vi "dotNET SSL Socket.vi"() -> ()   [LabVIEW 2013]
uses:
  dotNET SSL Socket/dotNET SSL Server/dotNET SSL Server.lvclass
  dotNET SSL Socket/dotNET SSL Listener/dotNET Listener.lvclass
panel:
  out "error out":errorcluster
  in  "stop":bool
  out "string":string
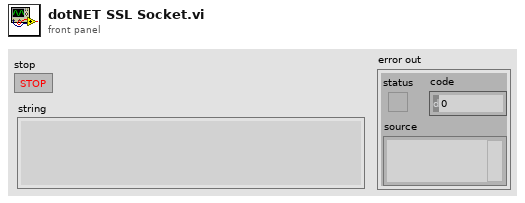
[diagram p1: front panel]
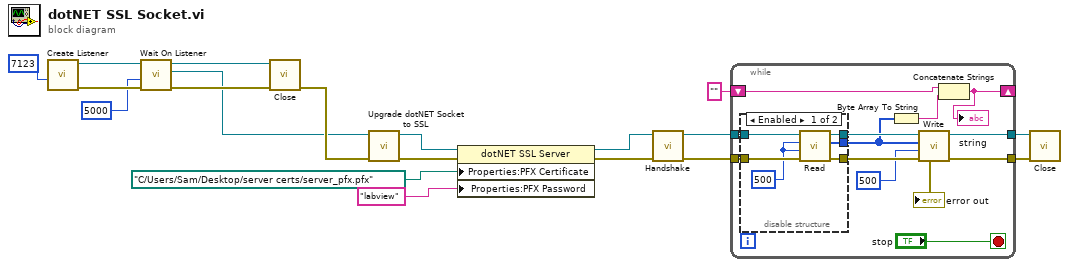
[diagram p0: block diagram]
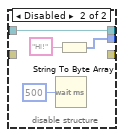
[diagram p2: hidden frame]
diagram:
  n1 = call-dynamic "Create Listener.vi"("timeout ms (5000)"=7123 ("port")) -> ("error out"=w15:errorcluster, "dotNET Listener out"=w14:refnum<class "dotNET Listener.lvclass">)  [unwired: 9 in]
  n2 = call-dynamic "Wait On Listener.vi"("error in (no error)"=w15, "timeout ms (5000)"=5000, "dotNET Listener in"=w14) -> ("error out"=w11:errorcluster, "Socket out"=w3:refnum<class "Socket.lvclass">, "dotNET Listener out"=w13:refnum<class "dotNET Listener.lvclass">)  [unwired: 6 in]
  n3 = call-dynamic "Close.vi"("error in (no error)"=w11, "dotNET Listener in"=w13) -> ("error out"=w10:errorcluster)  [unwired: 9 in]
  n4 = call "Upgrade dotNET Socket to SSL.vi"("error in (no error)"=w10, "Socket in"=w3) -> ("error out"=w9:errorcluster, "dotNET SSL Socket out"=w7:refnum<class "dotNET SSL Server.lvclass">)  [unwired: 8 in]
  n5 = property class="dotNET SSL Server"(reference=w7, error in=w9, "Properties:PFX Certificate"=path "C:/Users/Sam/Desktop/server certs/server_pfx.pfx", "Properties:PFX Password"="labview" ("password")) -> (reference out=w6:refnum<class "dotNET SSL Server.lvclass">, error out=w8:errorcluster)
  n6 = call-dynamic "Handshake.vi"("error in (no error)"=w8, "dotNET SSL Socket in"=w6) -> ("error out"=w2:errorcluster, "dotNET SSL Socket out"=w1:refnum<class "dotNET SSL Server.lvclass">)  [unwired: 8 in]
  n7 = while {
    tunnel: w2 -> [w31]
    tunnel: w1 -> [w29]
    tunnel: [w24] -> w18
    tunnel: [w25] -> w19
    shift-right: [w20] -> _
    shift-left: "" -> [w21]
    stop <- "stop" stop-if-true
    n8 = disable-structure shown="Enabled" {
      disable-tunnel: w31 -> [w37 _]
      disable-tunnel: [w36 _] -> w30
      disable-tunnel: w29 -> [w35 w41]
      disable-tunnel: [w33 w41] -> w28
      disable-tunnel: [w32 w39] -> w26
      frame Enabled {
        w34 = 500 ("timeout ms (25000)")
        n9 = call-dynamic "Read.vi"("error in (no error)"=w37, "timeout ms (5000)"=w34, "# bytes to read"=w34, "dotNET SSL Socket in"=w35) -> ("error out"=w36:errorcluster, "Read Bytes"=w32:u8[], "dotNET SSL Socket out"=w33:refnum<class "dotNET SSL Server.lvclass">)  [unwired: 5 in]
      }
      frame Disabled {
        n10 = Wait (ms)(milliseconds to wait=u32 500) -> ()  [unwired: 1 out]
        n11 = String To Byte Array(string="Hi!") -> (unsigned byte array=w39:u8[])
      }
    }
    n12 = Byte Array To String(unsigned byte array=w26) -> (string=w22:string)
    n13 = call-dynamic "Write.vi"("error in (no error)"=w30, "timeout ms (5000)"=500 ("timeout ms (25000)"), "Bytes to write"=w26, "dotNET SSL Socket in"=w28) -> ("error out"=w24:errorcluster, "dotNET SSL Socket out"=w25:refnum<class "dotNET SSL Server.lvclass">)  [unwired: 5 in, 1 out]
    "error out" <- w24
    n14 = Concatenate Strings(w21, w22) -> (w20:string)
    "string" <- w20
  }
  n15 = call-dynamic "Close.vi"("error in (no error)"=w18, "dotNET SSL Socket in"=w19) -> ()  [unwired: 9 in, 1 out]
